vi "Water Tank KC.vi"() -> ()   [LabVIEW 2018]
panel:
  in  "Main Tank Set Level":dbl
  in  "Tank #2 Set Level":dbl
  in  "Temp Set Value":dbl
  in  "Tank #1 Set Level":dbl
  in  "E Stop":bool
  in  "Reset":bool
  in  "start":bool
  in  "Auto/Manual":bool
  out "Pos #2":bool
  out "Pos #1":bool
  in  "Heater":bool
  in  "Conveyor":bool
  in  "Pump":bool
  in  "Fill \nCup #2":bool
  in  "Fill \nCup #1":bool
  in  "Fill \nTank #2":bool
  in  "Fill \nTank #1":bool
  out "Tank #2 Temp":dbl(slide) scale=0.0..150.0
  out "Main Tank Level":dbl(slide) scale=0.0..20.0
  out "Alerts":string
  out "Filling \nCup #2":bool
  out "Filling \nCup #1":bool
  out "Filling \nTank #2":bool
  out "Filling \nTank #1":bool
  out "Tank #1 Level":dbl(slide) scale=0.0..20.0
  out "Tank #2 Level":dbl(slide) scale=0.0..20.0
  out "Status":string
  in  "stop":bool
  out "Heater":bool
  out "Conv on":bool
  out "Pump on":bool
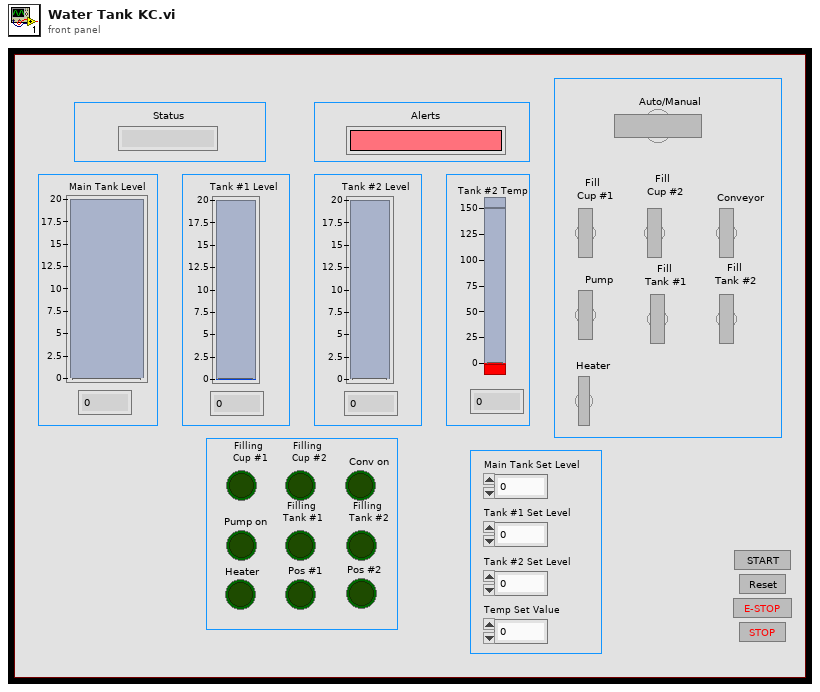
[diagram p1: front panel]
types:
  T1 = enum16{"Sate 0 Home", "State 1 Checking Main Tank", "State 2 Filling Tanks #1 & #2", "State 3 Moving to Position #1", "State 4 FillIng Cup #1 ", "State 5 Moving to Position #2", "State 6 Heating Tank #2", "State 7 Filling Cup #2", "State 8 Shutdown", "Manual"}
  T2 = cluster{"data[0]":bool, "data[1]":bool, "data[2]":bool, "data[3]":bool, "data[4]":bool, "data[5]":bool, "data[6]":bool, "data[7]":bool, "data[8]":bool}
  T3 = cluster{"Fill \nTank #1":bool, "Fill \nTank #2":bool, "Fill \nCup #1":bool, "Fill \nCup #2":bool, bool, "Pump":bool, "Conveyor":bool, "Heater":bool}
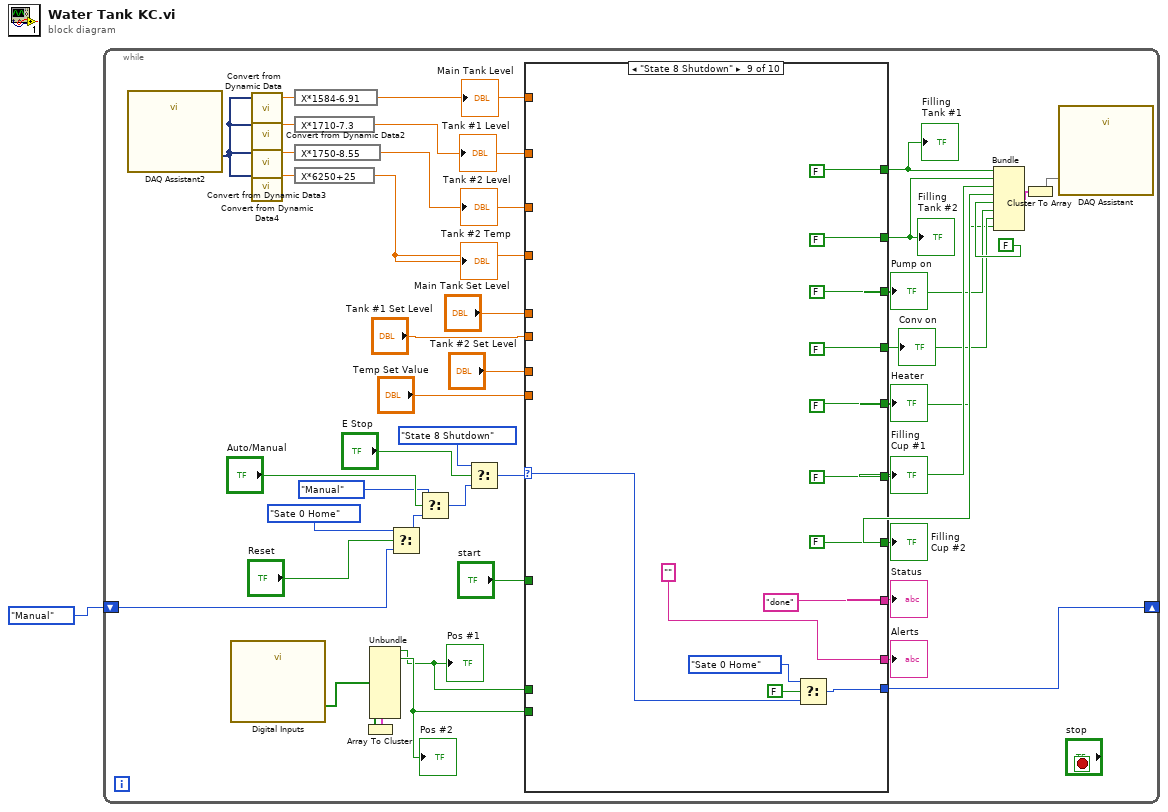
[diagram p0: block diagram]
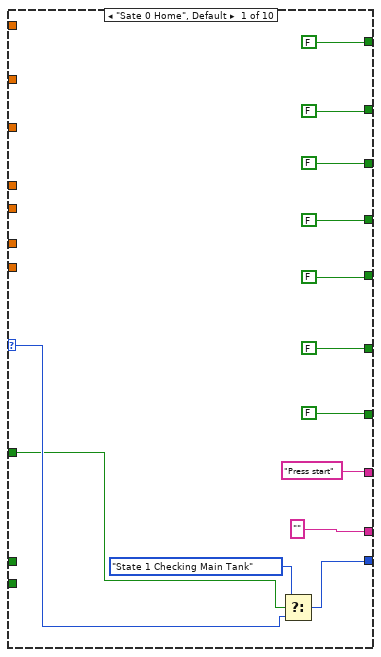
[diagram p2: hidden frame]
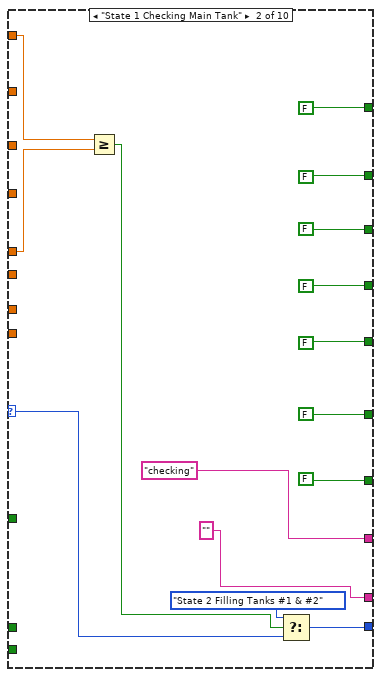
[diagram p3: hidden frame]
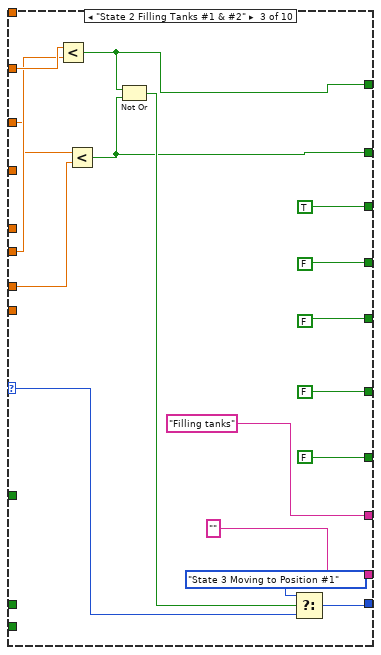
[diagram p4: hidden frame]
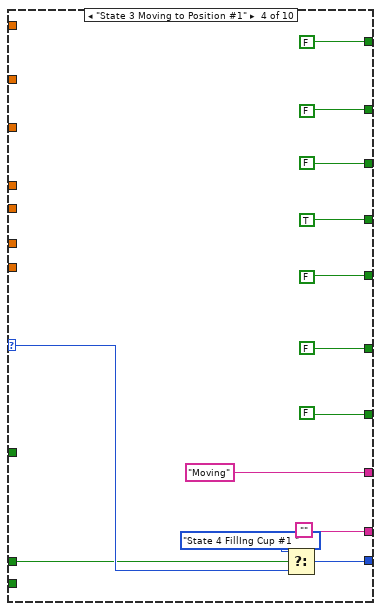
[diagram p5: hidden frame]
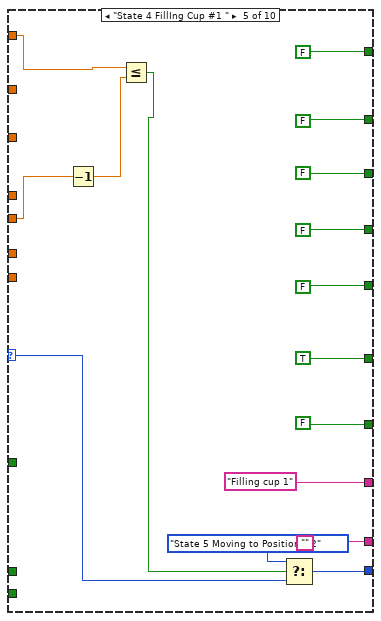
[diagram p6: hidden frame]
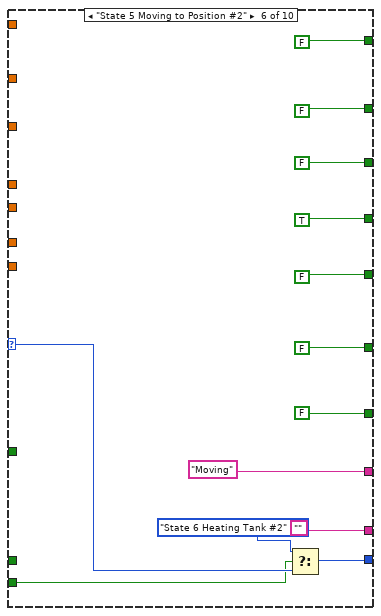
[diagram p7: hidden frame]
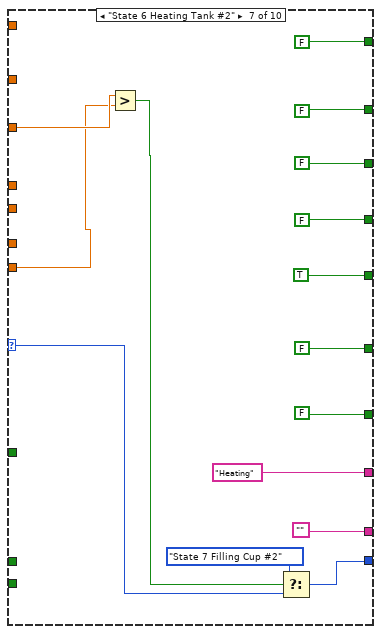
[diagram p8: hidden frame]
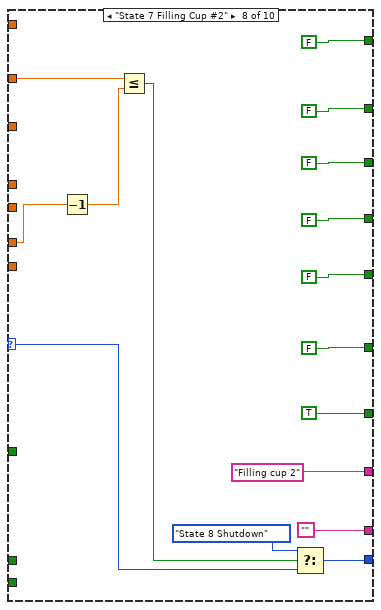
[diagram p9: hidden frame]
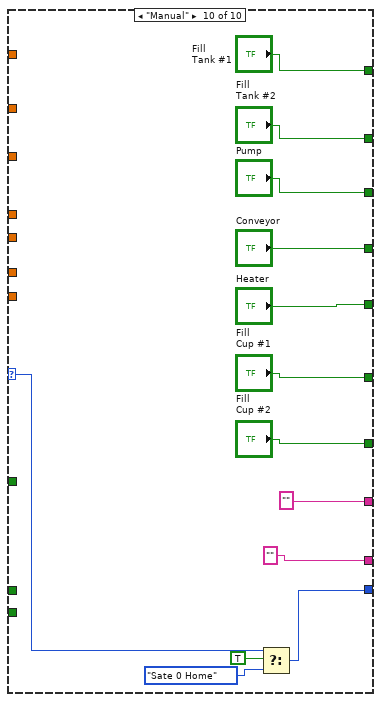
[diagram p10: hidden frame]
diagram:
  n1 = while {
    shift-right: [w40] -> _
    shift-left: T1."Manual" -> [w10]
    stop <- "stop" stop-if-true
    n2 = call "DAQ Assistant2"() -> ("data"=w20:dynamicdata)  [unwired: 17 in, 2 out]
    n3 = call "Digital Inputs"() -> ("data"=w31:bool[])  [unwired: 17 in, 2 out]
    n4 = call "Convert from Dynamic Data"("Dynamic Data Type"=w20) -> ("Scalar"=w32:dbl)  [unwired: 3 in]
    n5 = call "Convert from Dynamic Data2"("Dynamic Data Type"=w20) -> ("Scalar"=w39:dbl)  [unwired: 3 in]
    n6 = call "Convert from Dynamic Data3"("Dynamic Data Type"=w20) -> ("Scalar"=w38:dbl)  [unwired: 3 in]
    n7 = call "Convert from Dynamic Data4"("Dynamic Data Type"=w20) -> ("Scalar"=w34:dbl)  [unwired: 3 in]
    n8 = expression code="X*1584-6.91"(w32) -> (w37:dbl)
    "Main Tank Level" <- w37
    n9 = expression code="X*1710-7.3"(w39) -> (w36:dbl)
    "Tank #1 Level" <- w36
    n10 = expression code="X*1750-8.55"(w38) -> (w35:dbl)
    "Tank #2 Level" <- w35
    n11 = expression code="X*6250+25"(w34) -> (w33:dbl)
    "Tank #2 Temp" <- w33
    n12 = Array To Cluster(array=w31) -> (cluster=w41:T2)
    n13 = Unbundle(w41) -> ("data[0]"=w14:bool, "data[1]"=w15:bool)  [unwired: 7 out]
    "Pos #1" <- w14
    "Pos #2" <- w15
    n14 = Select(t=T1."Sate 0 Home", s="Reset", f=w10) -> (s? t:f=w9:T1)
    n15 = Select(t=T1."Manual", s="Auto/Manual", f=w9) -> (s? t:f=w6:T1)
    n16 = Select(t=T1."State 8 Shutdown", s="E Stop", f=w6) -> (s? t:f=w5:T1)
    n17 = case shown="\"State 8 Shutdown\"" w5 {
      selector: w5 -> [w47 w58 w81 w91 w107 w120 w136 w151 w164 w185]
      tunnel: ["Press start" "checking" "Filling tanks" "Moving" "Filling cup 1" "Moving" "Heating" "Filling cup 2" "done" ""] -> w42
      tunnel: [FALSE FALSE FALSE FALSE TRUE FALSE FALSE FALSE FALSE "Fill \nCup #1"] -> w28
      tunnel: [FALSE FALSE FALSE FALSE FALSE FALSE TRUE FALSE FALSE "Heater"] -> w23
      tunnel: [FALSE FALSE FALSE TRUE FALSE TRUE FALSE FALSE FALSE "Conveyor"] -> w24
      tunnel: [FALSE FALSE TRUE FALSE FALSE FALSE FALSE FALSE FALSE "Pump"] -> w25
      tunnel: [FALSE FALSE w73 FALSE FALSE FALSE FALSE FALSE FALSE "Fill \nTank #1"] -> w30
      tunnel: [FALSE FALSE w72 FALSE FALSE FALSE FALSE FALSE FALSE "Fill \nTank #2"] -> w29
      tunnel: [FALSE FALSE FALSE FALSE FALSE FALSE FALSE TRUE FALSE "Fill \nCup #2"] -> w27
      tunnel: [w48 w63 w82 w92 w108 w121 w137 w152 w165 w186] -> w40
      tunnel: w37 -> [_ w61 _ _ _ _ _ _ _ _]
      tunnel: w36 -> [_ _ w78 _ w104 _ _ _ _ _]
      tunnel: w35 -> [_ _ w76 _ _ _ _ w148 _ _]
      tunnel: w33 -> [_ _ _ _ _ _ w133 _ _ _]
      tunnel: "Main Tank Set Level" -> [_ w60 _ _ _ _ _ _ _ _]
      tunnel: "Tank #2 Set Level" -> [_ _ w75 _ _ _ _ w149 _ _]
      tunnel: "Tank #1 Set Level" -> [_ _ w77 _ w105 _ _ _ _ _]
      tunnel: "Temp Set Value" -> [_ _ _ _ _ _ w132 _ _ _]
      tunnel: w15 -> [_ _ _ _ _ w118 _ _ _ _]
      tunnel: w14 -> [_ _ _ w89 _ _ _ _ _ _]
      tunnel: "start" -> [w44 _ _ _ _ _ _ _ _ _]
      tunnel: ["" "" "" "" "" "" "" "" "" ""] -> w2
      frame "Sate 0 Home", Default {
        n18 = Select(t=T1."State 1 Checking Main Tank", s=w44, f=w47) -> (s? t:f=w48:T1)
      }
      frame "State 1 Checking Main Tank" {
        n19 = Greater Or Equal?(x=w61, y=w60) -> (x >= y?=w59:bool)
        n20 = Select(t=T1."State 2 Filling Tanks #1 & #2", s=w59, f=w58) -> (s? t:f=w63:T1)
      }
      frame "State 2 Filling Tanks #1 & #2" {
        n21 = Less?(x=w78, y=w77) -> (x < y?=w73:bool)
        n22 = Less?(x=w76, y=w75) -> (x < y?=w72:bool)
        n23 = Not Or(1:w72, 2:w73) -> (0:w74:bool)
        n24 = Select(t=T1."State 3 Moving to Position #1", s=w74, f=w81) -> (s? t:f=w82:T1)
      }
      frame "State 3 Moving to Position #1" {
        n25 = Select(t=T1."State 4 FillIng Cup #1 ", s=w89, f=w91) -> (s? t:f=w92:T1)
      }
      frame "State 4 FillIng Cup #1 " {
        n26 = Decrement(x=w105) -> (x-1=w102:dbl)
        n27 = Less Or Equal?(x=w104, y=w102) -> (x <= y?=w103:bool)
        n28 = Select(t=T1."State 5 Moving to Position #2", s=w103, f=w107) -> (s? t:f=w108:T1)
      }
      frame "State 5 Moving to Position #2" {
        n29 = Select(t=T1."State 6 Heating Tank #2", s=w118, f=w120) -> (s? t:f=w121:T1)
      }
      frame "State 6 Heating Tank #2" {
        n30 = Greater?(x=w133, y=w132) -> (0:w131:bool)
        n31 = Select(t=T1."State 7 Filling Cup #2", s=w131, f=w136) -> (s? t:f=w137:T1)
      }
      frame "State 7 Filling Cup #2" {
        n32 = Decrement(x=w149) -> (x-1=w147:dbl)
        n33 = Less Or Equal?(x=w148, y=w147) -> (x <= y?=w146:bool)
        n34 = Select(t=T1."State 8 Shutdown", s=w146, f=w151) -> (s? t:f=w152:T1)
      }
      frame "State 8 Shutdown" {
        n35 = Select(t=T1."Sate 0 Home", s=FALSE, f=w164) -> (s? t:f=w165:T1)
      }
      frame "Manual" {
        n36 = Select(t=w185, s=TRUE, f=T1."Sate 0 Home") -> (s? t:f=w186:T1)
      }
    }
    "Pump on" <- w25
    "Conv on" <- w24
    "Heater" <- w23
    "Status" <- w42
    "Filling \nTank #1" <- w30
    "Filling \nCup #1" <- w28
    "Filling \nCup #2" <- w27
    "Filling \nTank #2" <- w29
    "Alerts" <- w2
    n37 = Bundle("Fill \nTank #1"=w30, "Fill \nTank #2"=w29, "Fill \nCup #1"=w28, "Fill \nCup #2"=w27, FALSE, "Pump"=w25, "Conveyor"=w24, "Heater"=w23) -> (w22:T3)  [unwired: 1 in]
    n38 = Cluster To Array(cluster=w22) -> (array=w21:bool[])
    n39 = call "DAQ Assistant"("data"=w21) -> ()  [unwired: 17 in, 2 out]
  }
